vi "PointOverlayV1.vi"(8 "Point":i32[](array[numeric]), 9 "Count":i32, 11 "Image1":T1) -> (3 "Image1 Out":T1)   [LabVIEW 2017]
uses:
  <vilib>/vision/Image Controls.llb/IMAQ Image.ctl
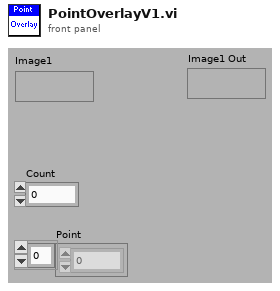
[diagram p1: front panel]
types:
  T1 = typedef "IMAQ Image.ctl" = refnum<image>
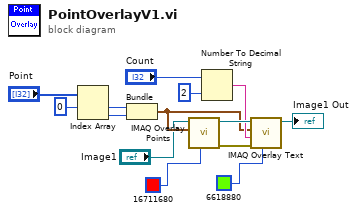
[diagram p0: block diagram]
diagram:
  n1 = Index Array(array="Point", index #1=0 ("index")) -> (element #1=w7:i32, element #2=w6:i32)  [unwired: 1 in]
  n2 = Bundle(w7, w6) -> (w8:cluster{i32, i32})  [unwired: 1 in]
  n3 = call "IMAQ Overlay Points"("Color"=u32 16711680, "Point"=w8, "Image"="Image1") -> ("error out"=w12:errorcluster, "Image Out"=w13:T1)  [unwired: 7 in]
  n4 = Number To Decimal String(number="Count", width (-)=i16 2) -> (decimal integer string=w9:string)
  n5 = call "IMAQ Overlay Text"("Text Color (black)"=u32 6618880, "error in (no error)"=w12, "String"=w9, "Origin"=w8, "Image"=w13) -> ("Image Out"=→"Image1 Out":T1)  [unwired: 5 in, 1 out]
